vi "Host_PulsehistogramSimple.vi"() -> ()   [LabVIEW 2012]
uses:
  <vilib>/FPGAPlugInAG/PXIe-7962R/niLvFpga_Open_PXIe-7962R.vi
  <vilib>/rvi/interface/common/dynamic/niFpgaDynamicAddResources.vi
  <vilib>/Utility/error.llb/Error Cluster From Error Code.vi
  <vilib>/rvi/errors/niLvFpgaAdjustHostInterfaceError.vi
  <vilib>/FPGAPlugInAG/Dynamic/niLvFpga_Close_Dynamic.vi
  <vilib>/rvi/interface/nirviOpenFPGA/nirviOpenFPGA.xnode
  FPGA Bitfiles/PulsehistogramSimple_NI5771.lvbitx
  <vilib>/rvi/interface/nirviReadWriteControl/nirviReadWriteControl.xnode
  <vilib>/rvi/interface/nirviMethod/nirviMethod.xnode
  <vilib>/rvi/interface/nirviCloseFPGA/nirviCloseFPGA.xnode
  NiFpgaLv.dll
  <vilib>/rvi/interface/Simulation/niFpgaSimulationCallBeginRW.vi
  <vilib>/Analysis/NI_AALPro.lvlib
  <vilib>/FPGAPlugInAG/Dynamic/niLvFpga_ReadFifo_Dynamic.vi
  <vilib>/rvi/errors/niLvFpgaMergeErrorWithErrorCode.vi
panel:
  out "ToHostU8FIFO Overflow":bool
  in  "Baseline":u8
  out "Laser pulse length histogram":T1(graph)
  out "Laser graph":waveform(i16)(graph)
  out "Laser pulse interval histogram":T1(graph)
  out "Channel 0 relative histogram":u64[](graph)
  out "Channel 0 graph":waveform(u8)(graph)
  out "Loop counter":i32
  out "ToHostU64FIFO Overflow":bool
  out "error out":errorcluster
  out "Channel 0 histogram":T1(graph)
  out "Configured?":bool
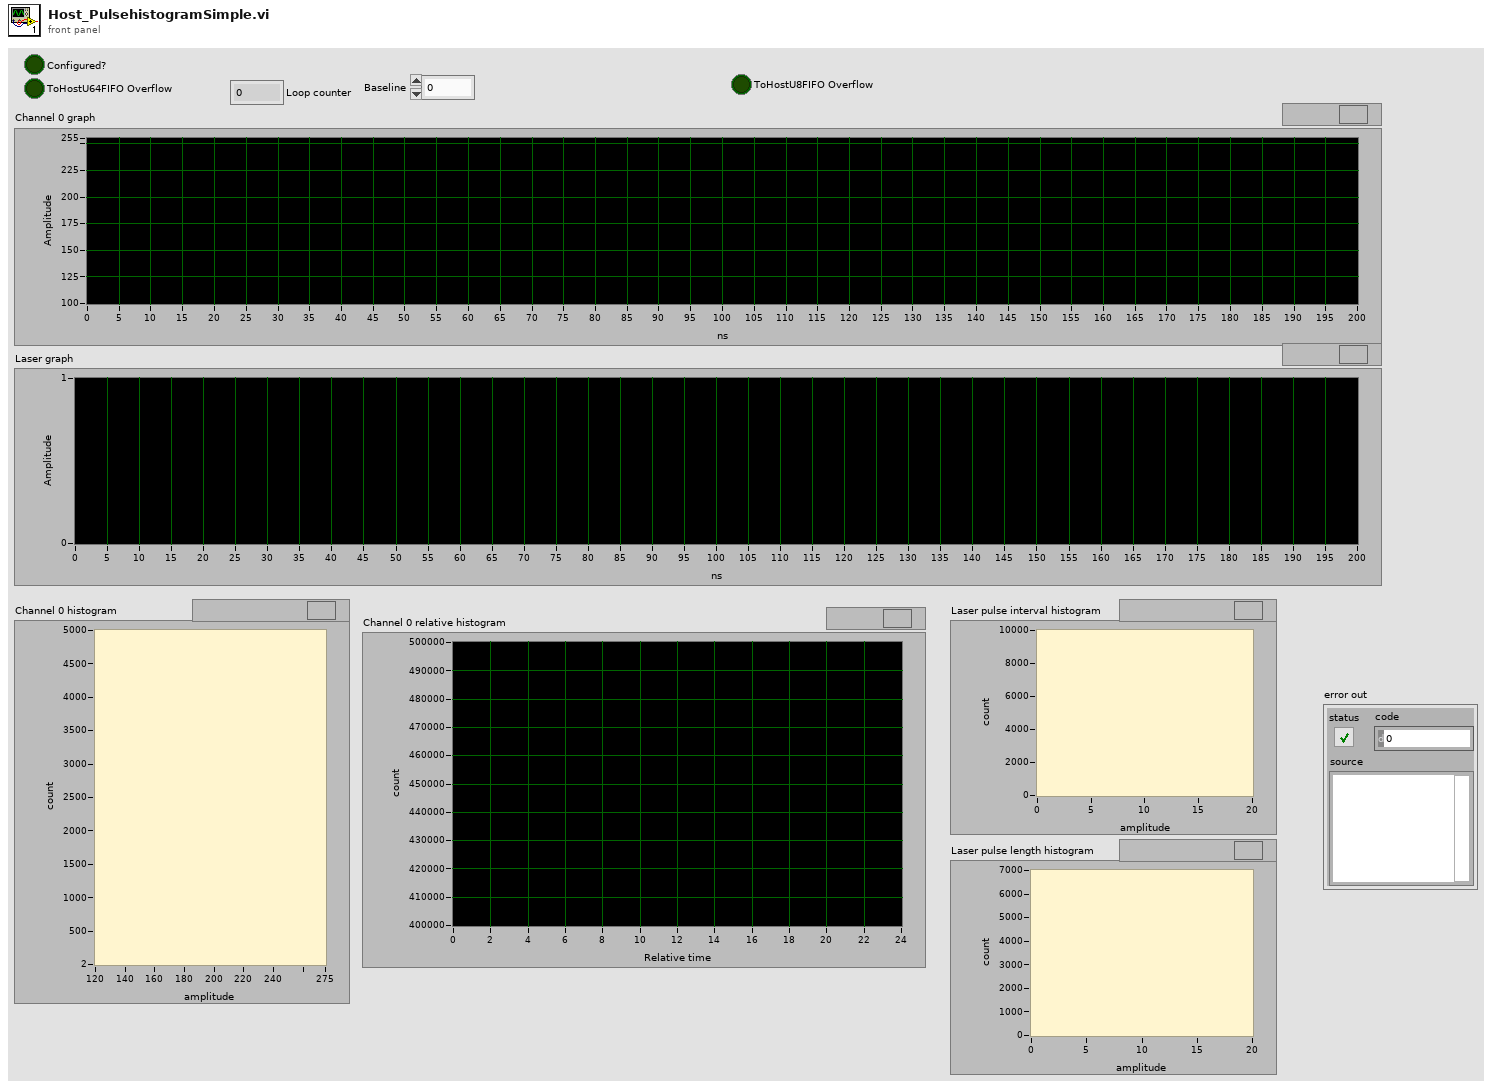
[diagram p1: front panel]
types:
  T1 = cluster{"X Values":dbl[], "Histogram: h(x)":i32[]}
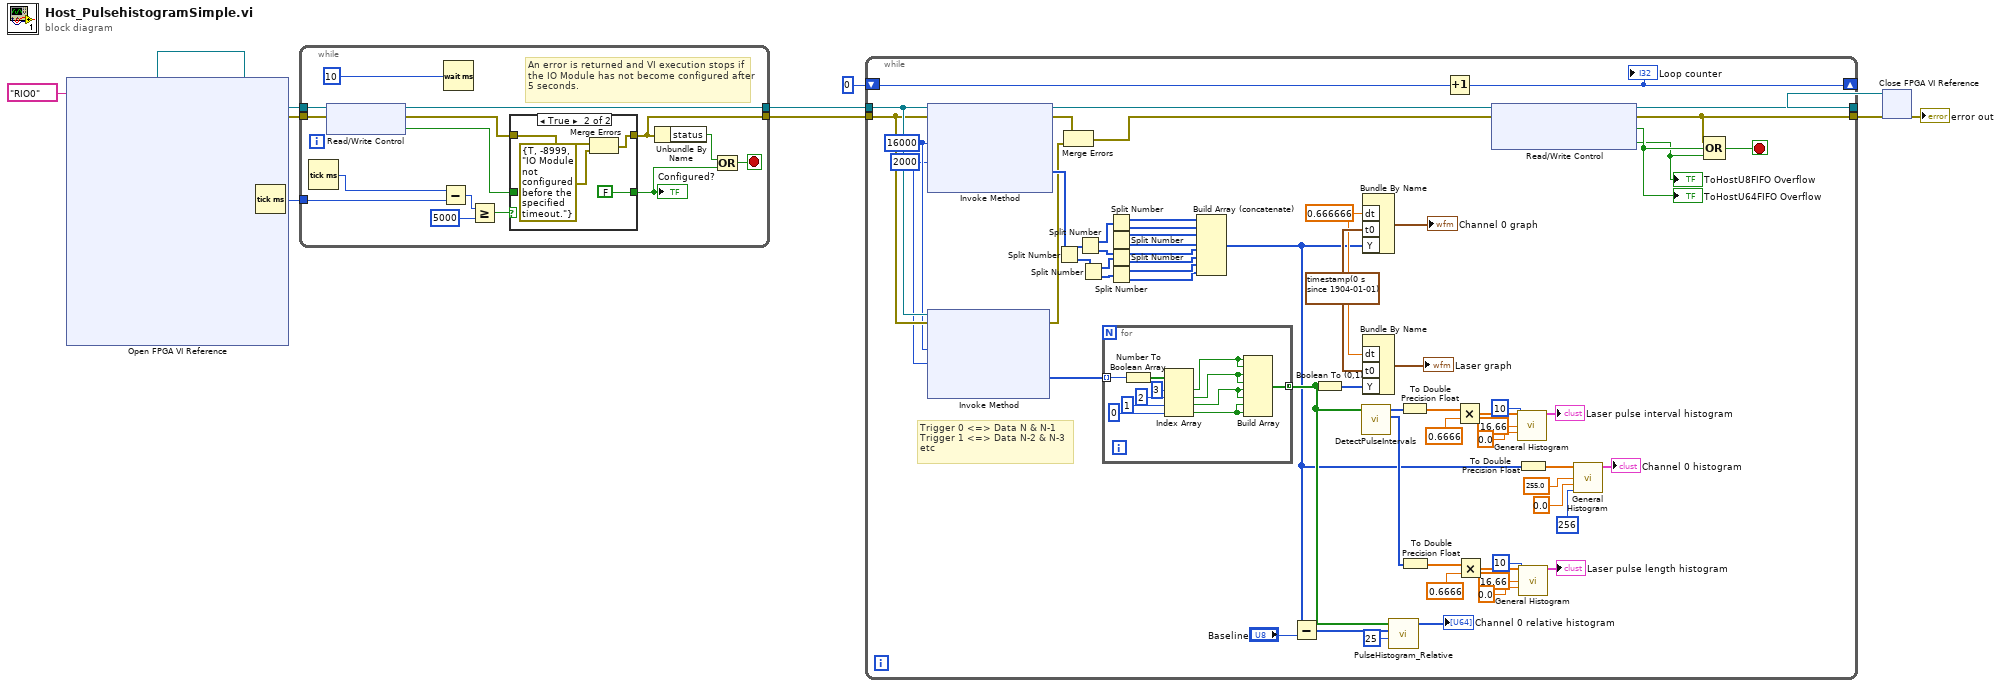
[diagram p0: block diagram]
diagram:
  n1 = xnode "Open FPGA VI Reference"("resource name"=tag "RIO0") -> ("FPGA VI Reference Out"=w1:refnum<k20>, "error out"=w4:errorcluster)  [unwired: 1 in]
  n2 = Tick Count (ms)() -> (millisecond timer value=w9:u32)
  n3 = while {
    tunnel: w4 -> [w18]
    tunnel: [w22] -> w3
    tunnel: [w14] -> w2
    tunnel: w1 -> [w17]
    tunnel: w9 -> [w12]
    stop <- w20 stop-if-true
    # "An error is returned and VI execution stops if the IO Module has not become configured after 5 seconds."
    n4 = Tick Count (ms)() -> (millisecond timer value=w13:u32)
    n5 = xnode "Read/Write Control"("FPGA VI Reference In"=w17, "error in"=w18) -> ("FPGA VI Reference Out"=w14:refnum<k20>, "error out"=w15:errorcluster, "Configured?"=w16:bool)
    n6 = Subtract(x=w13, y=w12) -> (x-y=w11:u32)
    n7 = Wait (ms)(milliseconds to wait=u32 10) -> ()  [unwired: 1 out]
    n8 = Greater Or Equal?(x=w11, y=u32 5000) -> (x >= y?=w23:bool)
    n9 = case shown="True" w23 {
      tunnel: [w27 FALSE ("Configured?")] -> w19
      tunnel: w16 -> [w27 _]
      tunnel: [w26 w30] -> w22
      tunnel: w15 -> [w26 w28]
      frame False {
      }
      frame True {
        n10 = Merge Errors(w28, errorcluster {"status"=TRUE, "code"=-8999, "source"="IO Module not configured before the specified timeout."} ("error in")) -> (w30:errorcluster)
      }
    }
    "Configured?" <- w19
    n11 = Unbundle By Name(w22) -> ("status"=w21:bool)
    n12 = Or(x=w21, y=w19) -> (x .or. y?=w20:bool)
  }
  n13 = while {
    tunnel: w3 -> [w71]
    tunnel: w2 -> [w72]
    tunnel: [w92] -> w8
    tunnel: [w93] -> w7
    shift-right: [w88] -> _
    shift-left: 0 -> [w89]
    stop <- w90 stop-if-true
    w63 = 0.666666 ("dt")
    w68 = timestamp(0 s since 1904-01-01) ("t0")
    w69 = 2000 ("Timeout (ms)")
    w70 = u32 16000 ("Number of Elements")
    # "Trigger 0 <=> Data N & N-1\nTrigger 1 <=> Data N-2 & N-3\netc"
    n14 = xnode "Invoke Method"("FPGA VI Reference In"=w72, "error in"=w71, "Number of Elements"=w70, "Timeout (ms)"=w69) -> ("FPGA VI Reference Out"=w94:refnum<k20>, "error out"=w33:errorcluster, "Data"=w87:u64[])  [unwired: 1 out]
    n15 = xnode "Invoke Method"("FPGA VI Reference In"=w72, "error in"=w71, "Number of Elements"=w70, "Timeout (ms)"=w69) -> ("error out"=w34:errorcluster, "Data"=w62:u8[])  [unwired: 2 out]
    n16 = Split Number(x=w87) -> (hi(x)=w86:u32[], lo(x)=w85:u32[])
    n17 = Merge Errors(w33, w34) -> (w32:errorcluster)
    n18 = Split Number(x=w86) -> (hi(x)=w84:u16[], lo(x)=w83:u16[])
    n19 = Split Number(x=w85) -> (hi(x)=w82:u16[], lo(x)=w81:u16[])
    n20 = for {
      tunnel: w62 -> [w105] mode=indexing
      tunnel: [w95] -> w60 mode=concatenating
      n21 = Number To Boolean Array(number=w105) -> (Boolean array=w104:bool[])
      n22 = Index Array(array=w104, index #1=3 ("index"), index #2=2 ("index"), index #3=1 ("index"), index #4=0 ("index")) -> (element #1=w99:bool, element #2=w98:bool, element #3=w97:bool, element #4=w96:bool)
      n23 = Build Array(w99, w99, w98, w98, w97, w97, w96, w96) -> (w95:bool[])
    }
    n24 = Split Number(x=w84) -> (hi(x)=w80:u8[], lo(x)=w79:u8[])
    n25 = Split Number(x=w83) -> (hi(x)=w78:u8[], lo(x)=w77:u8[])
    n26 = Split Number(x=w82) -> (hi(x)=w76:u8[], lo(x)=w75:u8[])
    n27 = Split Number(x=w81) -> (hi(x)=w74:u8[], lo(x)=w73:u8[])
    n28 = Build Array (concatenate)(w80, w79, w78, w77, w76, w75, w74, w73) -> (w38:u8[])
    n29 = Subtract(x=w38, y="Baseline") -> (x-y=w37:u8[])
    n30 = Boolean To (0,1)(Boolean=w60) -> (0, 1=w61:i16[])
    n31 = call "DetectPulseIntervals.vi"("Binary array probe"=w60) -> ("Pulse lenghts out"=w39:i32[], "Interflank intervals out"=w57:i32[])  [unwired: 8 in, 1 out]
    n32 = Bundle By Name("dt"=w63, "t0"=w68, "Y"=w38) -> (→"Channel 0 graph":waveform(u8))  [unwired: 1 in]
    n33 = Bundle By Name("dt"=w63, "t0"=w68, "Y"=w61) -> (→"Laser graph":waveform(i16))  [unwired: 1 in]
    n34 = call "PulseHistogram_Relative.vi"("No of SI bins"=25, "U8 array probe"=w37, "Binary array reference"=w60) -> ("Histogram"=→"Channel 0 relative histogram":u64[])  [unwired: 8 in]
    n35 = To Double Precision Float(number=w57) -> (double precision float=w56:dbl[])
    n36 = To Double Precision Float(number=w39) -> (double precision float=w46:dbl[])
    n37 = Increment(x=w89) -> (x+1=w88:i32)
    "Loop counter" <- w88
    n38 = Multiply(x=w56, y=0.6666) -> (x*y=w54:dbl[])
    n39 = Multiply(x=w46, y=0.6666) -> (x*y=w44:dbl[])
    n40 = xnode "Read/Write Control"("FPGA VI Reference In"=w94, "error in"=w32) -> ("FPGA VI Reference Out"=w93:refnum<k20>, "error out"=w92:errorcluster, "ToHostU64FIFO Overflow"=w91:bool, "ToHostU8FIFO Overflow"=w35:bool)
    "ToHostU64FIFO Overflow" <- w91
    "ToHostU8FIFO Overflow" <- w35
    n41 = call <vilib>:"General Histogram.vi"("X"=w54, "max"=16.66, "min"=0.0, "# bins"=10) -> ("Histogram Graph"=→"Laser pulse interval histogram":T1)  [unwired: 7 in, 4 out]
    n42 = call <vilib>:"General Histogram.vi"("X"=w44, "max"=16.66, "min"=0.0, "# bins"=10) -> ("Histogram Graph"=→"Laser pulse length histogram":T1)  [unwired: 7 in, 4 out]
    n43 = To Double Precision Float(number=w38) -> (double precision float=w58:dbl[])
    n44 = call <vilib>:"General Histogram.vi"("X"=w58, "max"=255.0, "min"=0.0, "# bins"=256) -> ("Histogram Graph"=→"Channel 0 histogram":T1)  [unwired: 7 in, 4 out]
    n45 = Compound Arithmetic op=OR(w92, w91, w35) -> (w90:bool)
  }
  n46 = xnode "Close FPGA VI Reference"("FPGA VI Reference In"=w7, "error in"=w8) -> ("error out"=→"error out":errorcluster)
